vi "Get Image Data From PictureBox.vi"(8 "error in (no error)":errorcluster, 11 "Image":refnum<k24>) -> (0 "error out":errorcluster, 2 "Image Data":T1, 3 "Image Out":refnum<k24>)   [LabVIEW 2014]
doc: "This VI will output the <b>Image Data</b> for a given <b>PictureBox</b> .NET object that has an image loaded into it."
uses:
  <vilib>/picture/picture.llb/imagedata.ctl
  System.Drawing
  <vilib>/wsapi/NI_WebServices.lvlib
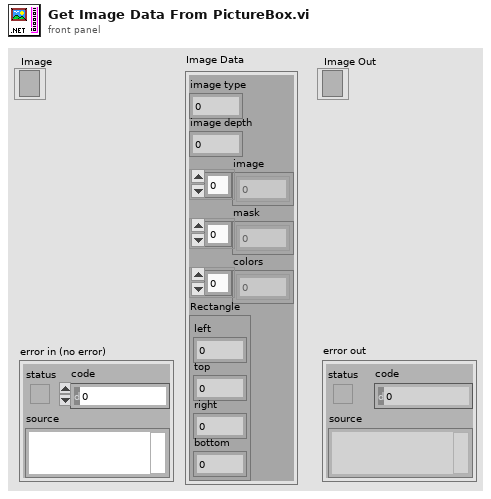
[diagram p1: front panel]
types:
  T1 = typedef "imagedata.ctl" = cluster{"image type":i32, "image depth":i32, "image":u8[], "mask":u8[], "colors":u32[], "Rectangle":cluster{"left":i16, "top":i16, "right":i16, "bottom":i16}}
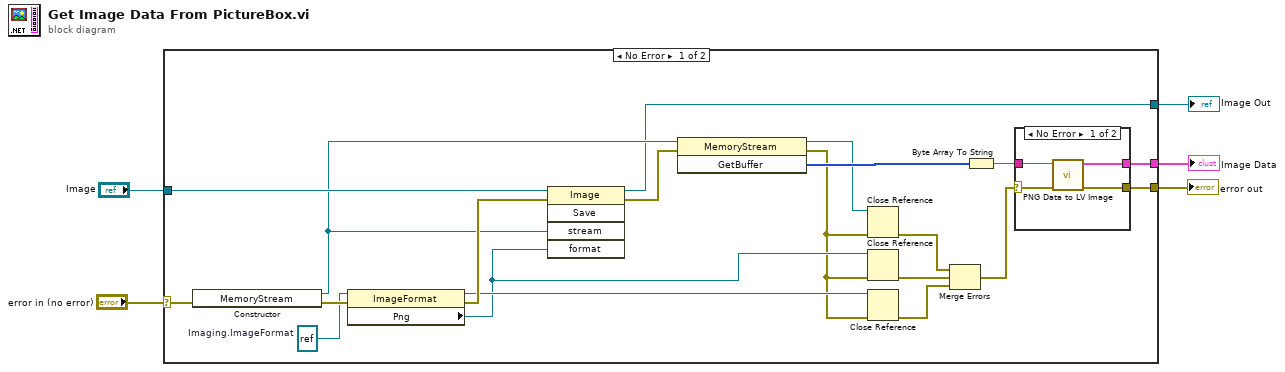
[diagram p0: block diagram]
diagram:
  n1 = case shown="No Error" "error in (no error)" {
    selector: "error in (no error)" -> [w6 w32]
    tunnel: [w20 w32] -> w5
    tunnel: [w19 _] -> w4
    tunnel: "Image" -> [w10 w31]
    tunnel: [w7 w31] -> w2
    frame No Error {
      w12 = refnum<k24> refnum  # Imaging.ImageFormat
      n2 = constructor class="MemoryStream"(error in=w6) -> (reference out=w9:refnum<k24>, error out=w23:errorcluster)  [unwired: 2 in, 1 out]
      n3 = property class="ImageFormat"(reference=w12, error in=w23) -> (reference out=w18:refnum<k24>, error out=w22:errorcluster, "Png"=w16:refnum<k24>)
      n4 = invoke class="Image" method="Save"(reference=w10, error in=w22, "stream"=w9, "format"=w16) -> (reference out=w7:refnum<k24>, error out=w21:errorcluster)  [unwired: 1 in, 3 out]
      n5 = invoke class="MemoryStream" method="GetBuffer"(reference=w9, error in=w21) -> (reference out=w17:refnum<k24>, error out=w13:errorcluster, "GetBuffer"=w25:u8[])  [unwired: 1 in]
      n6 = Close Reference(reference=w17, error in (no error)=w13) -> (error out=w8:errorcluster)
      n7 = Close Reference(reference=w16, error in (no error)=w13) -> (error out=w14:errorcluster)
      n8 = Close Reference(reference=w18, error in (no error)=w13) -> (error out=w15:errorcluster)
      n9 = Merge Errors(w8, w14, w15) -> (w11:errorcluster)
      n10 = Byte Array To String(unsigned byte array=w25) -> (string=w24:string)
      n11 = case shown="No Error" w11 {
        selector: w11 -> [w26 w30]
        tunnel: w24 -> [w29 _]
        tunnel: [w28 w30] -> w20
        tunnel: [w27 _] -> w19
        frame No Error {
          n12 = call <vilib>:"PNG Data to LV Image.vi"("error in (no error)"=w26, "png data"=w29) -> ("error out"=w28:errorcluster, "image data"=w27:T1)  [unwired: 8 in]
        }
        frame Error {
        }
      }
    }
    frame Error {
    }
  }
  "error out" <- w5
  "Image Data" <- w4
  "Image Out" <- w2
